vi "Global 2.vi"() -> ()   [LabVIEW 2012]
panel:
  in  "Array":dbl[][](array[numeric])
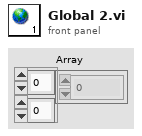
[diagram p1: front panel]
diagram:
